vi "Globalne_zmienne.vi"() -> ()   [LabVIEW 2022 SP3]
panel:
  in  "Ustronianka":dbl
  in  "UstalonaCena4":dbl
  in  "UstalonaCena3":dbl
  in  "UstalonaCena2":dbl
  in  "UstalonaCena1":dbl=1.4256114757235e-311
  out "Cena 12":dbl
  out "Cena 11":dbl
  out "Cena 10":dbl
  out "Cena 9":dbl
  out "Cena 8":dbl
  out "Cena 7":dbl=1.4256114754706e-311
  in  "Tarczyn":dbl
  in  "Tiger":dbl
  in  "Black":dbl
  in  "Muszynianka":dbl
  in  "Tymbark":dbl
  in  "Cappy":dbl
  in  "Nestea":dbl
  in  "Mountain Dew":dbl
  in  "Kofola":dbl
  in  "Pepsi":dbl
  in  "Coca-Cola":dbl
  out "Cena 6":dbl
  out "Cena 5":dbl
  out "Cena 4":dbl
  out "Cena 3":dbl
  out "Cena 2":dbl
  out "Cena":dbl
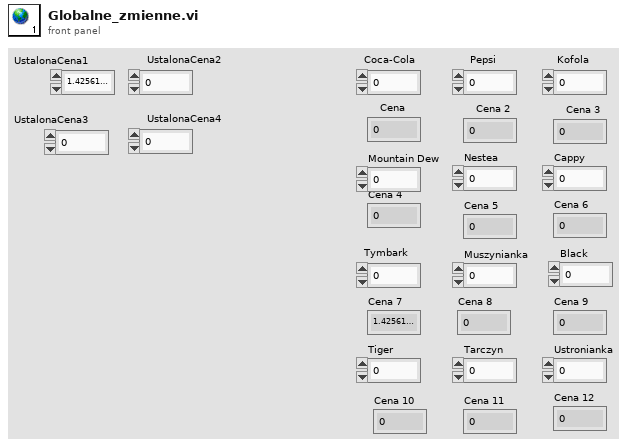
[diagram p1: front panel]
diagram:
